vi "Write Tx Values and Read Rx Values Until Equal.vi"(6 "Tx values":dbl[](array[numeric]), 7 "timeout (1000 ms)":i32=1000, 8 "error in":errorcluster, 9 "Rx aliases":string[](array[string]), 10 "Tx aliases":string[](array[string]), 11 "workspace manager in":T1) -> (0 "error out":errorcluster, 2 "values equal":bool, 3 "workspace manager out":T1)   [LabVIEW 2017, in "VeriStandTestUtilities.lvlib"]
uses:
  <vilib>/NI Veristand/Execution/Workspace/WorkspaceAPI.ctl
  NationalInstruments.VeriStand.ClientAPI
  <vilib>/NI Veristand/Execution/Workspace/NI VeriStand - Set Multiple Channel Values.vi
  VeriStandTestUtilities.lvlib
  <vilib>/NI VeriStand/Execution/Workspace/NI_VS Workspace ExecutionAPI.lvlib
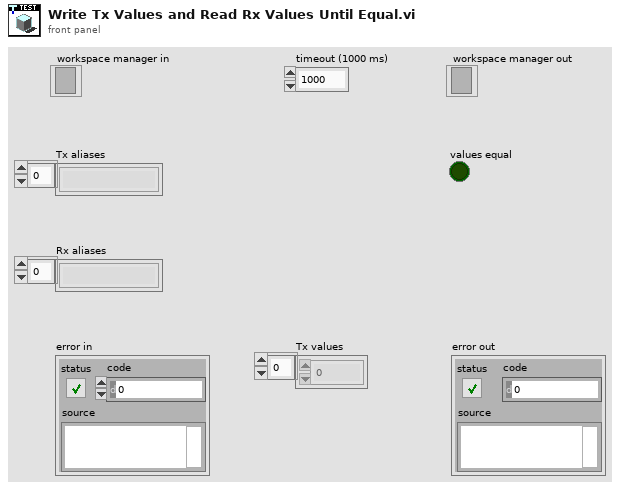
[diagram p1: front panel]
types:
  T1 = typedef "NI_VS Workspace ExecutionAPI.lvlib/WorkspaceAPI.ctl" = refnum<k24>
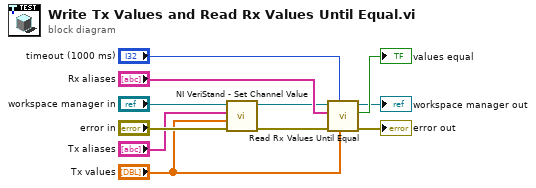
[diagram p0: block diagram]
diagram:
  n1 = call-poly <vilib>:"NI VeriStand - Set Channel Value.vi"("error in (no error)"="error in", "Values"="Tx values", "Channels"="Tx aliases", "WorkspaceManager in"="workspace manager in") -> ("error out"=w5:errorcluster, "WorkspaceManager out"=w6:T1)  [unwired: 6 in]
  n2 = call "Read Rx Values Until Equal.vi"("expected values"="Tx values", "timeout (1000 ms)"="timeout (1000 ms)", "error in"=w5, "Rx aliases"="Rx aliases", "workspace manager in"=w6) -> ("error out"=→"error out":errorcluster, "values equal expected"=→"values equal":bool, "workspace manager out"=→"workspace manager out":T1)  [unwired: 4 in]
